vi "Configure Loop Setup Parameters.vi"(0 "VISA resource name":refnum<visa-resource-name>, 1 "Unit Address (1)":u8=1, 5 "Channel 1 Control Type (0: Off)":u8(ring) items=["Off", "On/Off", "PID", "VPU", "VPB"], 7 "Channel 2 Control Type (0: Off)":u8(ring) items=["Off", "On/Off", "PID", "VPU", "VPB"], 9 "Control Action (True: Direct)":bool=TRUE, 11 "error in (no error)":errorcluster, 12 "Derivative Type (0: PV)":u8(ring) items=["PV", "Error"]) -> (4 "VISA resource name out":refnum<visa-resource-name>, 15 "error out":errorcluster)   [LabVIEW 2014, in "Eurotherm 35xx Series.lvlib"]
doc: "This VI configure Loop Setup parameters.\n\nDescription:\n\nOn/Off Control -\nOn/Off control is the simplest means of control but gives rise to fluctuations in the process variable. A degree of hysteresis or deadband must be set in On/Off control if the operation of the switching device is to be reduced and relay chatter is to be avoided.\nOn/Off control is a very simple form of control, which leads to oscillation of the process variable. This oscillation can affect the quality of the final product and is undesirable. The alternative is to use three term control, known as PID control.\n\nPID Control -\nPID or Three Term Control is an algorithm which controls the process to a setpoint. PID provides more stable control by continuously adjusting the output to compensate for the Error, the rate of change or the error and any continuous offsets.\nPID controllers must be tuned to the process they are controlling-\n-A too small proportional band gives temperature cycling (control loop instability). \n-A too large proportional band gives sluggish control, (a too feeble change of power in response to deviations of temperature). \n-A too small integral time will give an over eager response and result in instability. \n-A too large integral time will slow down both the approach to set point on a start up and return to set point after a disturbance. \n-Although derivative action helps to achieve stability a too large derivative time can also bring instability by an over eager power boost or throttle back. \n\nMotorised Valve Control-\nThe controller may be configured for motorised valve control as an alternative to the standard PID control algorithm. This algorithm is designed specifically for positioning motorised valves.\nThe control is performed by delivering open or close pulses in response to the control demand signal.\nThe motorised valve algorithm can operate in one of three ways:\n1. The so-called boundless mode, which does not require a position feedback potentiometer for control purposes; although one can be connected and used purely to display the valve’s position. \n2. Bounded, (or position), control mode, which requires a feedback potentiometer. This is closed-loop control determined by the valve’s position. \n\nWarning: This VI uses Controller Configuration Mode, this interrupts working process (device will not control).\nIt is recommended that the device should be disconnected from any active process."
uses:
  <instrlib>/Eurotherm 35xx Series/Eurotherm 35xx Series.lvlib
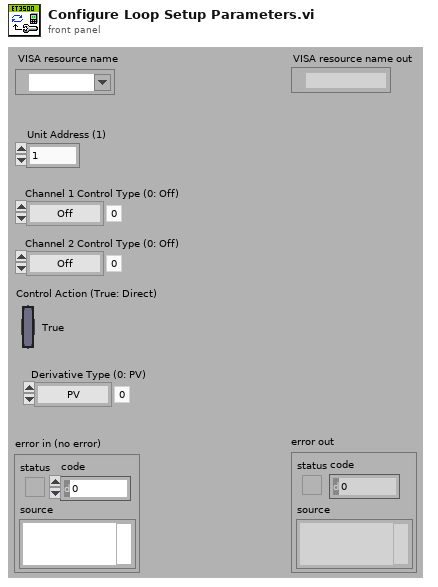
[diagram p1: front panel]
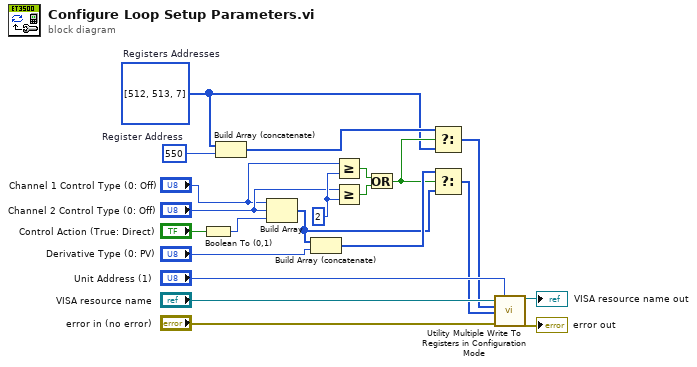
[diagram p0: block diagram]
diagram:
  w12 = u8 2 ("Register Addresses (0)")
  w16 = 550  # Register Address
  w3 = u16[] [512, 513, 7]  # Registers Addresses
  n1 = Boolean To (0,1)(Boolean="Control Action (True: Direct)") -> (0, 1=w14:i16)
  n2 = Build Array (concatenate)(w3, w16) -> (w4:i32[])
  n3 = Build Array("Channel 1 Control Type (0: Off)", "Channel 2 Control Type (0: Off)", w14) -> (w6:i16[])
  n4 = Build Array (concatenate)(w6, "Derivative Type (0: PV)") -> (w7:i16[])
  n5 = Greater Or Equal?(x="Channel 1 Control Type (0: Off)", y=w12) -> (x >= y?=w9:bool)
  n6 = Greater Or Equal?(x="Channel 2 Control Type (0: Off)", y=w12) -> (x >= y?=w8:bool)
  n7 = Or(x=w9, y=w8) -> (x .or. y?=w5:bool)
  n8 = Select(t=w4, s=w5, f=w3) -> (s? t:f=w1:i32[])
  n9 = Select(t=w7, s=w5, f=w6) -> (s? t:f=w2:i16[])
  n10 = call <instrlib>:"Utility Multiple Write To Registers in Configuration Mode.vi"("VISA resource name"="VISA resource name", "Unit Address (1)"="Unit Address (1)", "Registers Addresses (0)"=w1, "Data (0)"=w2, "error in (no error)"="error in (no error)") -> ("VISA resource name out"=→"VISA resource name out":refnum<visa-resource-name>, "error out"=→"error out":errorcluster)  [unwired: 9 in]
